vi "CustomBlinking.vi"() -> ()   [LabVIEW 2019]
uses:
  <vilib>/Utility/miscctls.llb/LVTextColorsTypeDef.ctl
panel:
  in  "Knob":dbl(knob) scale=0.0..1000.0
  in  "Numeric":dbl
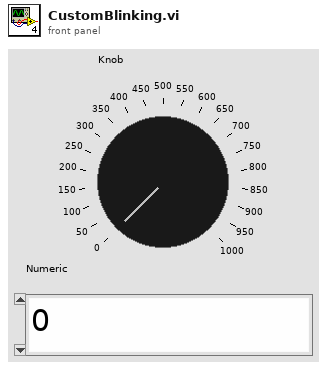
[diagram p1: front panel]
types:
  T1 = typedef "LVTextColorsTypeDef.ctl" = cluster{"Text Color":u32, "Background Color":u32}
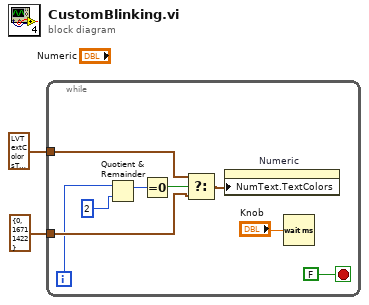
[diagram p0: block diagram]
diagram:
  n1 = while {
    tunnel: T1 {"Text Color"=16774656, "Background Color"=16720896} ("Numeric Text.Text Colors") -> [w8]
    tunnel: T1 {"Text Color"=0, "Background Color"=16711422} ("Numeric Text.Text Colors") -> [w7]
    i -> [w4]
    stop <- FALSE stop-if-true
    n2 = Quotient & Remainder(x=w4, y=2) -> (x-y*floor(x/y)=w5:i32)  [unwired: 1 out]
    n3 = Equal To 0?(x=w5) -> (x = 0?=w9:bool)
    n4 = Select(t=w8, s=w9, f=w7) -> (s? t:f=w6:T1)
    n5 = property on="Numeric" class="DigNum (strict)"("NumText.TextColors"=w6) -> ()  [unwired: 2 in, 2 out]
    n6 = Wait (ms)(milliseconds to wait="Knob") -> ()  [unwired: 1 out]
  }
